vi "newpoumiandatacomb.vi"(10 "columns":string[](array[string]), 11 "剖面数据":string[][](array[string])) -> (3 "结果字符串":string)   [LabVIEW 2016, in "212format_work.lvclass"]
uses:
  212format_work.lvclass
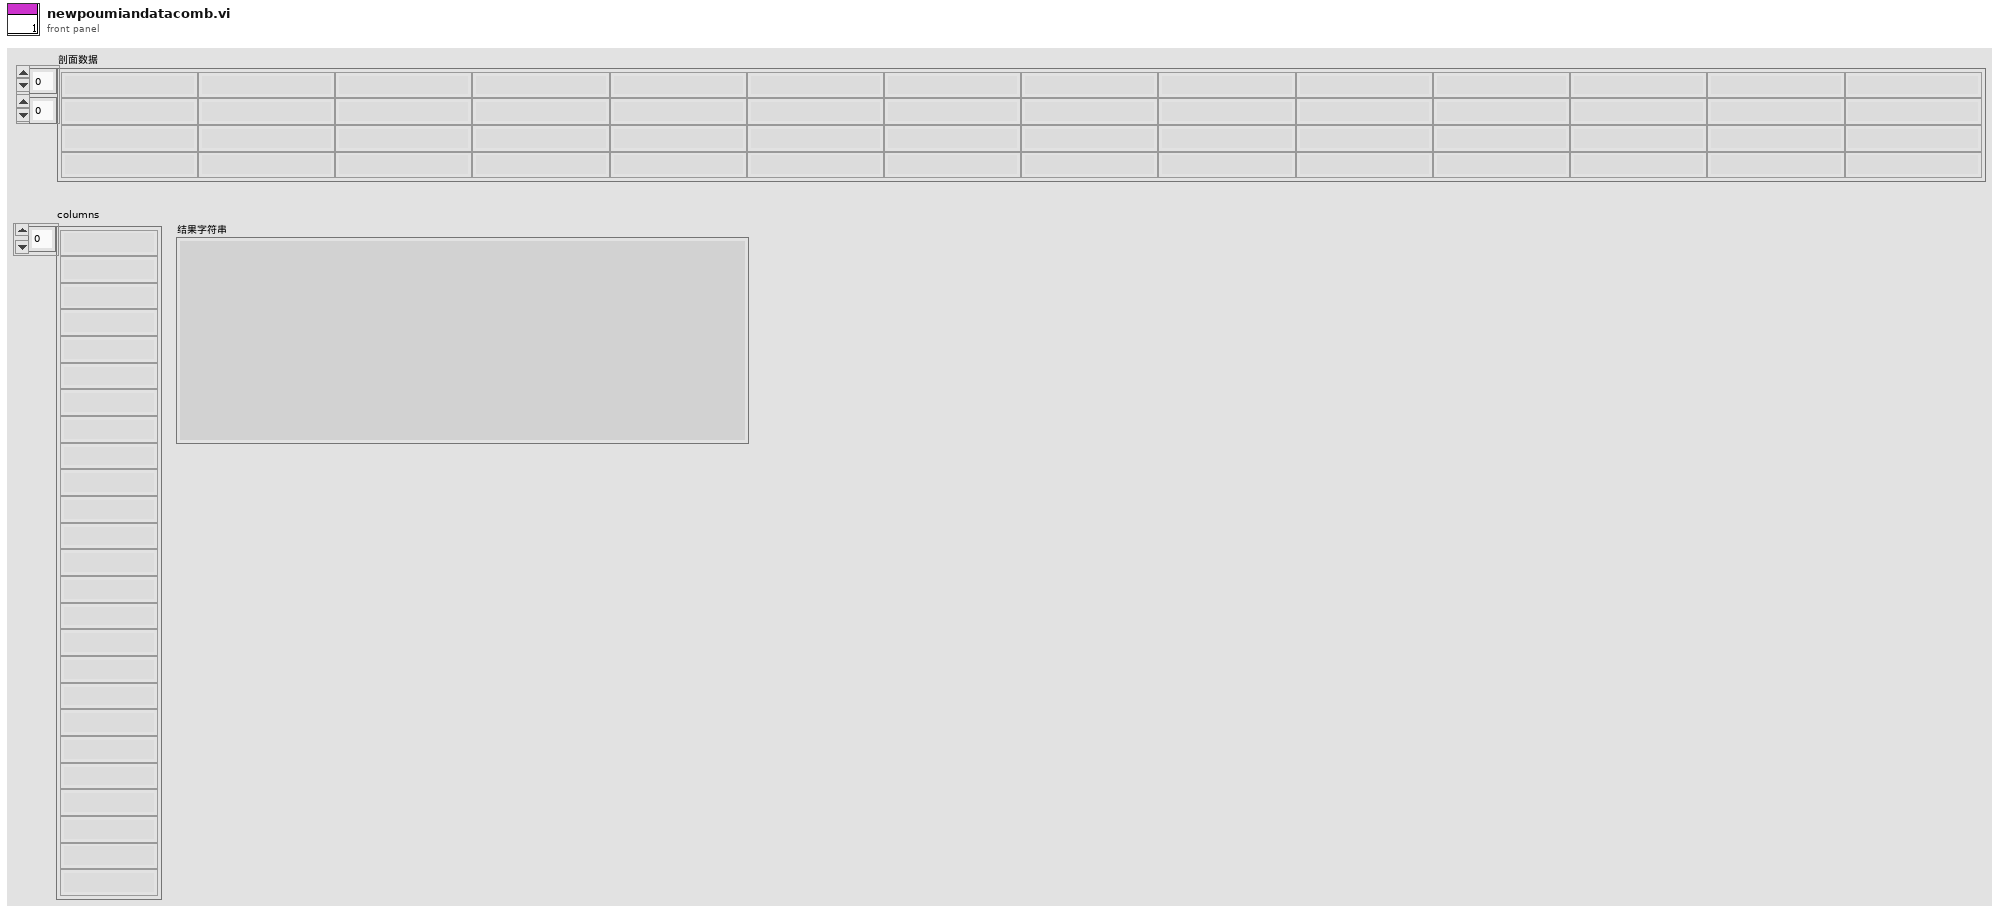
[diagram p1: front panel]
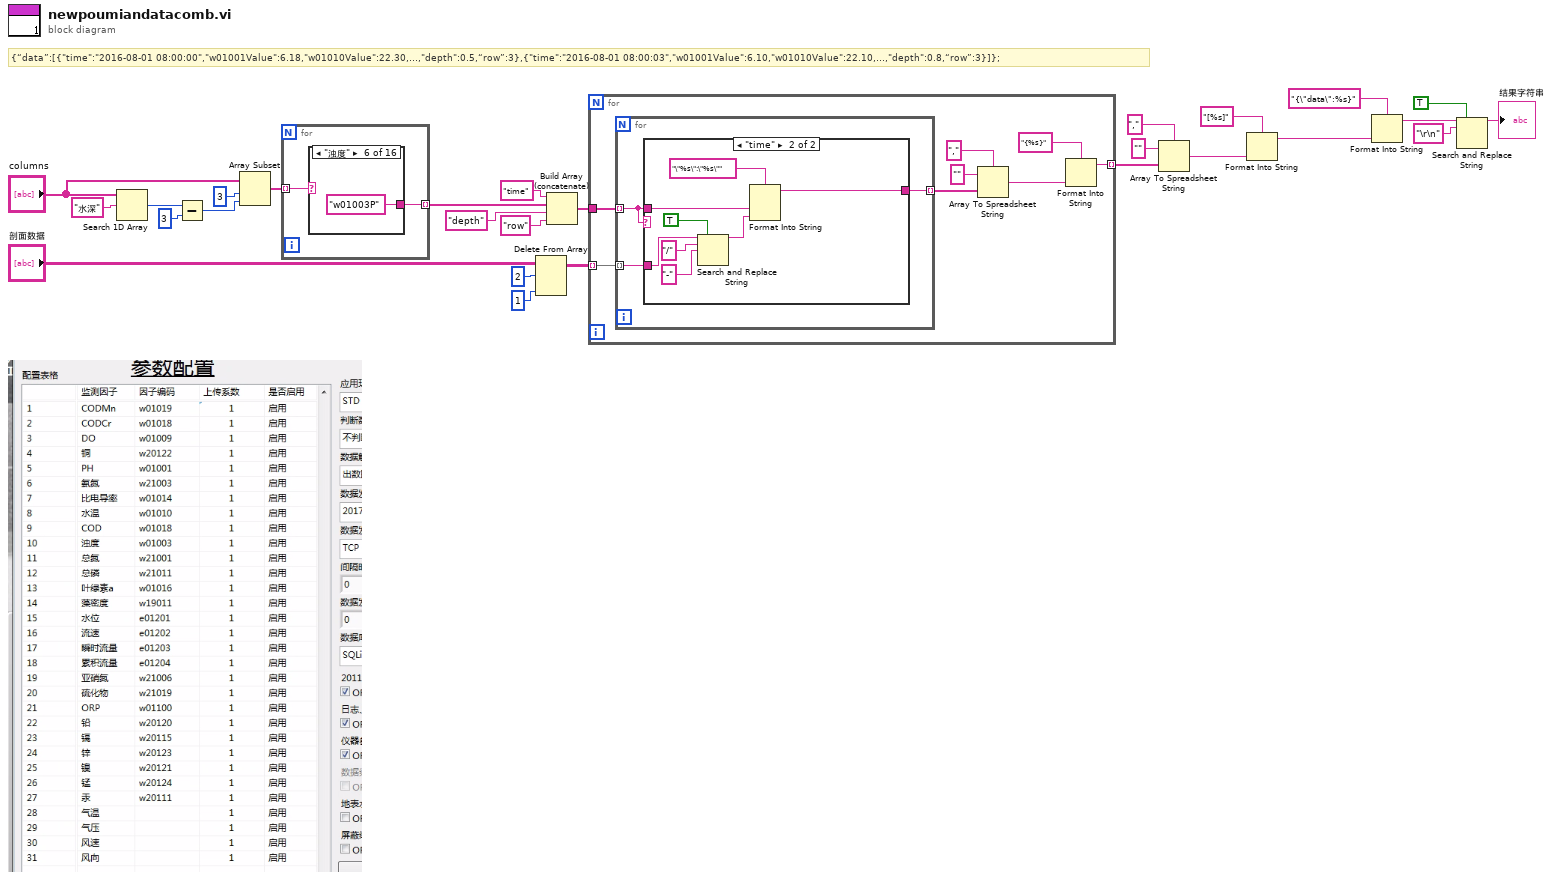
[diagram p0: block diagram]
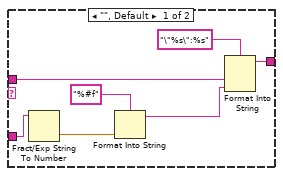
[diagram p2: hidden frame]
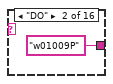
[diagram p4: hidden frame]
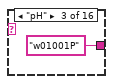
[diagram p5: hidden frame]
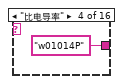
[diagram p6: hidden frame]
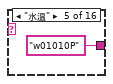
[diagram p7: hidden frame]
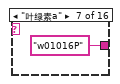
[diagram p8: hidden frame]
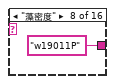
[diagram p9: hidden frame]
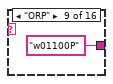
[diagram p10: hidden frame]
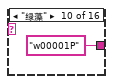
[diagram p11: hidden frame]
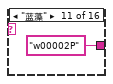
[diagram p12: hidden frame]
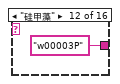
[diagram p13: hidden frame]
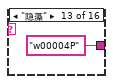
[diagram p14: hidden frame]
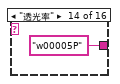
[diagram p15: hidden frame]
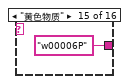
[diagram p16: hidden frame]
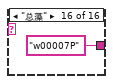
[diagram p17: hidden frame]
diagram:
  # "{“data”:[{\"time\":\"2016-08-01 08:00:00\",\"w01001Value\":6.18,\"w01010Value\":22.30,…,\"depth\":0.5,“row”:3},{\"time\":\"2016-08-01 08:00:03\",\"w01001Value\":6.10,\"w01010Value\":22.10,…,\"depth\":0.8,“row”:3}]};"
  n1 = Search 1D Array(1D array="columns", element="水深" ("元素")) -> (index of element=w17:i32)  [unwired: 1 in]
  n2 = Subtract(x=w17, y=3) -> (x-y=w23:i32)
  n3 = Array Subset(array="columns", index=3 ("索引"), length=w23) -> (w24:string[])
  n4 = for {
    tunnel: w24 -> [w29] mode=indexing
    tunnel: [w28] -> w21 mode=indexing
    n5 = case shown="\"浊度\"" w29 {
      tunnel: [_ "w01009P" "w01001P" "w01014P" "w01010P" "w01003P" "w01016P" "w19011P" "w01100P" "w00001P" "w00002P" "w00003P" "w00004P" "w00005P" "w00006P" "w00007P"] -> w28
      frame "", Default {
      }
      frame "DO" {
      }
      frame "pH" {
      }
      frame "比电导率" {
      }
      frame "水温" {
      }
      frame "浊度" {
      }
      frame "叶绿素a" {
      }
      frame "藻密度" {
      }
      frame "ORP" {
      }
      frame "绿藻" {
      }
      frame "蓝藻" {
      }
      frame "硅甲藻" {
      }
      frame "隐藻" {
      }
      frame "透光率" {
      }
      frame "黄色物质" {
      }
      frame "总藻" {
      }
    }
  }
  n6 = Delete From Array(array="剖面数据", length=2 ("长度"), index (col)=1 ("禁用的索引 (列)")) -> (array with subset deleted=w1:string[][])  [unwired: 1 in, 1 out]
  n7 = Build Array (concatenate)("time" ("元素"), w21, "depth" ("元素"), "row" ("元素")) -> (w20:string[])
  n8 = for {
    tunnel: w1 -> [w51] mode=indexing
    tunnel: w20 -> [w52]
    tunnel: [w46] -> w14 mode=indexing
    n9 = for {
      tunnel: w52 -> [w54] mode=indexing
      tunnel: w51 -> [w53] mode=indexing
      tunnel: [w55] -> w48 mode=indexing
      n10 = case shown="\"time\"" w54 {
        tunnel: [w61 w69] -> w55
        tunnel: w54 -> [w60 w68]
        tunnel: w53 -> [w58 w64]
        frame "", Default {
          n11 = Fract/Exp String To Number(string=w58) -> (number=w57:dbl)  [unwired: 3 in, 1 out]
          n12 = Format Into String(format string="%#f" ("格式字符串"), w57) -> (resulting string=w56:string)  [unwired: 2 in, 1 out]
          n13 = Format Into String(format string="\"%s\":%s" ("格式字符串"), w60, w56) -> (resulting string=w61:string)  [unwired: 2 in, 1 out]
        }
        frame "time" {
          n14 = Search and Replace String(replace all?=TRUE ("替换全部？(F)"), input string=w64, search string="/" ("搜索字符串"), replace string="-" ("替换字符串(\"\")")) -> (result string=w63:string)  [unwired: 4 in, 3 out]
          n15 = Format Into String(format string="\"%s\":\"%s\"" ("格式字符串"), w68, w63) -> (resulting string=w69:string)  [unwired: 2 in, 1 out]
        }
      }
    }
    n16 = Array To Spreadsheet String(delimiter (Tab)="," ("分隔符(Tab)"), array=w48, 3:"" ("格式字符串")) -> (spreadsheet string=w45:string)
    n17 = Format Into String(format string="{%s}" ("格式字符串"), w45) -> (resulting string=w46:string)  [unwired: 2 in, 1 out]
  }
  n18 = Array To Spreadsheet String(delimiter (Tab)="," ("分隔符(Tab)"), array=w14, 3:"" ("格式字符串")) -> (spreadsheet string=w10:string)
  n19 = Format Into String(format string="[%s]" ("格式字符串"), w10) -> (resulting string=w11:string)  [unwired: 2 in, 1 out]
  n20 = Format Into String(format string="{\"data\":%s}" ("格式字符串"), w11) -> (resulting string=w7:string)  [unwired: 2 in, 1 out]
  n21 = Search and Replace String(replace all?=TRUE ("替换全部？(F)"), input string=w7, search string="\r\n") -> (result string=→"结果字符串":string)  [unwired: 5 in, 3 out]
